vi "HW Configuration.vi"(8 "error in (no error)":errorcluster, 11 "Configuration in":refnum<class "Configuration.lvclass">) -> (0 "error out":errorcluster, 3 "Configuration out":refnum<class "Configuration.lvclass">)   [LabVIEW 2017, in "Hardware.lvlib" / "DAQ Configuration.lvclass"]
uses:
  DAQ/config/DAQ Configuration.lvclass
  <userlib>/Configuration Dialog Actor/Configuration.lvclass
  \\Mac\Home/Documents/Extensible-Config-Dialog/Configuration.lvclass
  DAQ/config/DAQ Configuration.lvclass/DAQ Configuration.ctl
panel:
  in  "Range":cluster{"Ranve (min)":dbl, "Range Max":dbl}
  in  "IO Channels":string="0:2"
  in  "Sample Rate":dbl
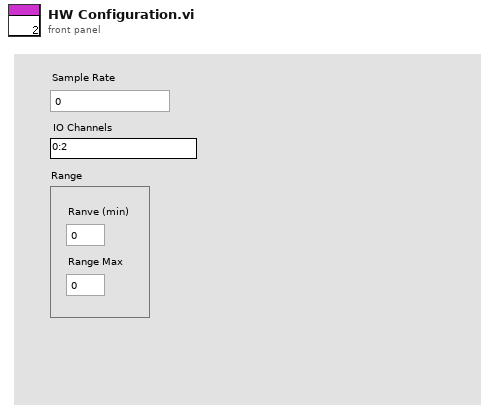
[diagram p1: front panel]
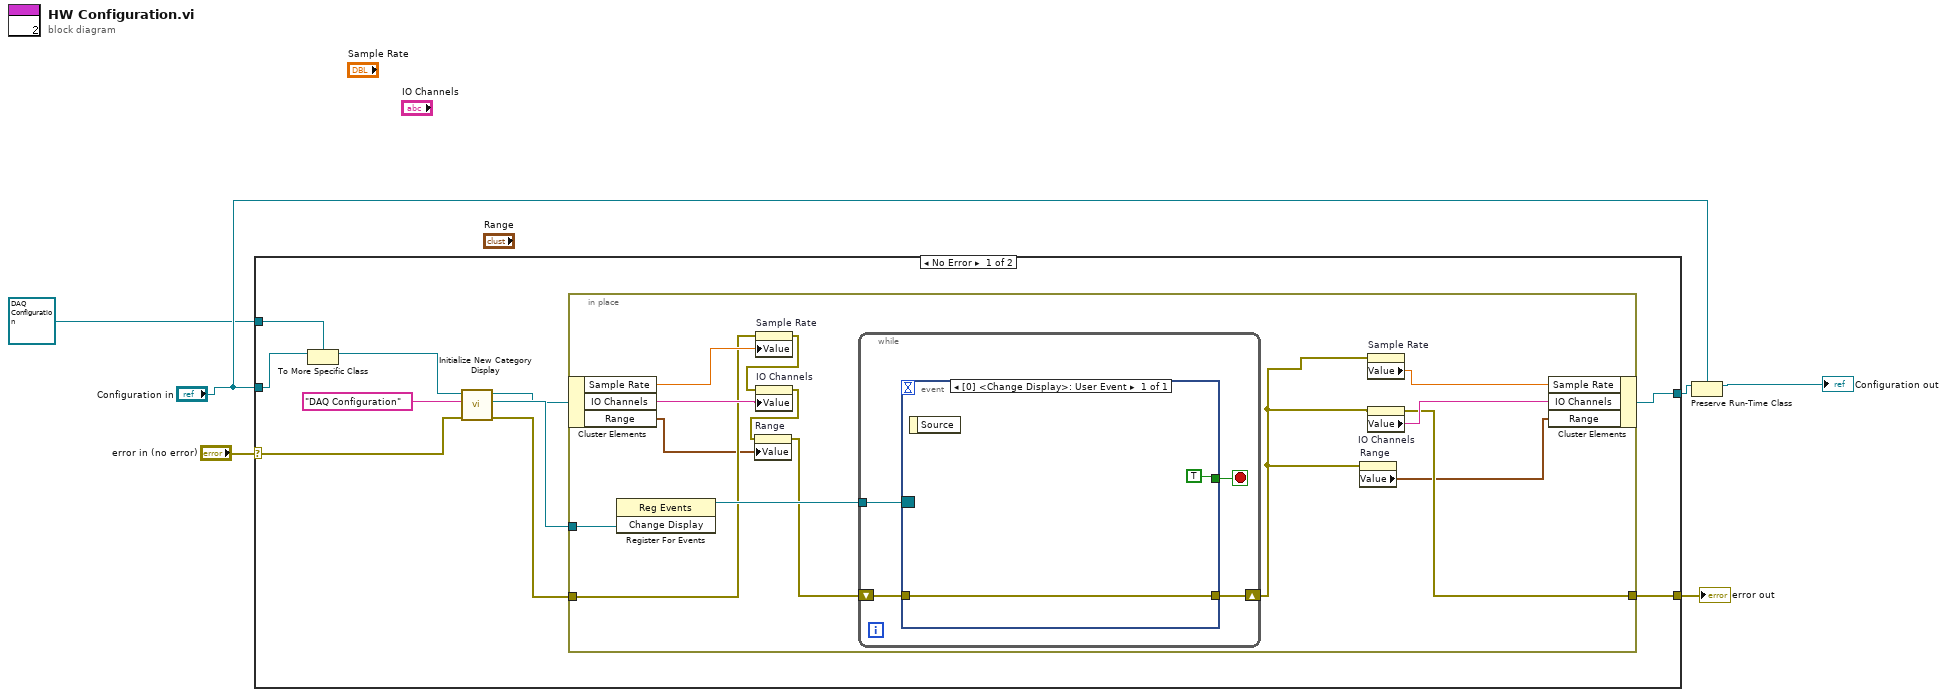
[diagram p0: block diagram]
diagram:
  n1 = case shown="No Error" "error in (no error)" {
    selector: "error in (no error)" -> [w12 w38]
    tunnel: [w11 w37] -> w3
    tunnel: [w14 w38] -> w6
    tunnel: "Configuration in" -> [w10 w37]
    tunnel: refnum<class "DAQ Configuration.lvclass"> refnum ("Hardware.lvlib:DAQ Configuration.lvclass") -> [w8 _]
    frame No Error {
      n2 = To More Specific Class(target class=w8, reference=w10) -> (specific class reference=w9:refnum<class "DAQ Configuration.lvclass">)  [unwired: 1 in, 1 out]
      n3 = call <userlib>:"Initialize New Category Display.vi"("error in (no error)"=w12, "Name to Display"="DAQ Configuration", "Configuration in"=w9) -> ("error out"=w15:errorcluster, "Change Display"=w16:refnum<user-event>, "Configuration Out"=w7:refnum<class "DAQ Configuration.lvclass">)  [unwired: 6 in]
      n4 = in-place {
        in-place-border: w16 -> [w30]
        in-place-border: w15 -> [w26]
        in-place-border: [w22] -> w14
        n5 = in-place-cluster #1(w7) -> ("Sample Rate"=w27:dbl, "IO Channels"=w28:string, "Range"=w21:cluster{"Ranve (min)":dbl, "Range Max":dbl})
        n6 = register-events(w30) -> (reference out=w29:refnum<event-registration>)  [unwired: 2 in, 1 out]
        n7 = property on="Sample Rate" class="DigNum (strict)"(error in=w26, "Value"=w27) -> (error out=w25:errorcluster)  [unwired: 1 in, 1 out]
        n8 = property on="IO Channels" class="Str"(error in=w25, "Value"=w28) -> (error out=w18:errorcluster)  [unwired: 1 in, 1 out]
        n9 = property on="Range" class="Clust (strict)"(error in=w18, "Value"=w21) -> (error out=w17:errorcluster)  [unwired: 1 in, 1 out]
        n10 = while {
          tunnel: w29 -> [w33]
          shift-right: [w32] -> w19
          shift-left: w17 -> [w31]
          stop <- w34 stop-if-true
          n11 = event shown="[0] <Change Display>: User Event" {
            selector: w33 -> [_]
            dyn-events: _ -> [_]
            timeout: _ -> [_]
            tunnel: [TRUE] -> w34
            tunnel: [w35] -> w32
            tunnel: w31 -> [w35]
            event User Event {
              n12 = event-data() -> ()  [unwired: 1 in, 1 out]
            }
          }
        }
        n13 = property on="Range" class="Clust (strict)"(error in=w19) -> ("Value"=w20:cluster{"Ranve (min)":dbl, "Range Max":dbl})  [unwired: 1 in, 2 out]
        n14 = property on="Sample Rate" class="DigNum (strict)"(error in=w19) -> ("Value"=w23:dbl)  [unwired: 1 in, 2 out]
        n15 = property on="IO Channels" class="Str"(error in=w19) -> (error out=w22:errorcluster, "Value"=w24:string)  [unwired: 1 in, 1 out]
        n16 = in-place-cluster #1("Sample Rate"=w23, "IO Channels"=w24, "Range"=w20) -> (w11:refnum<class "DAQ Configuration.lvclass">)
      }
    }
    frame Error {
    }
  }
  "error out" <- w6
  n17 = Preserve Run-Time Class(object in=w3, 2:"Configuration in") -> (object out=→"Configuration out":refnum<class "Configuration.lvclass">)  [unwired: 1 in, 1 out]
